vi "Main.vi"() -> ()   [LabVIEW 2012]
uses:
  SprayParams_Array.ctl
  ControlCore_Queue.ctl
  ControlCore_States.ctl
  <vilib>/DAQmx/write.llb/DAQmx Write (Digital Bool 1Line 1Point).vi
  <vilib>/DAQmx/miscellaneous.llb/DAQmx Fill In Error Info.vi
  <userlib>/Utility/ErrorLog_lib.lvlib
panel:
  out "ETF (min)":dbl format="%#.1g"
  out "Progress Bar":dbl(slide) scale=0.0..1.0
  out "String":string
  in  "STOP":bool
  in  "Close":bool
  in  "Open":bool
  in  "Start":bool
  out "Relay Status":bool
  in  "Spray Parameters":T1[](array[typedef])=[{"Cycle#"=20, "Spray Time"=1.25, "Dry Time"=15.0}] caption="Cycle#, Spray Time (s), Dry Time (s)"
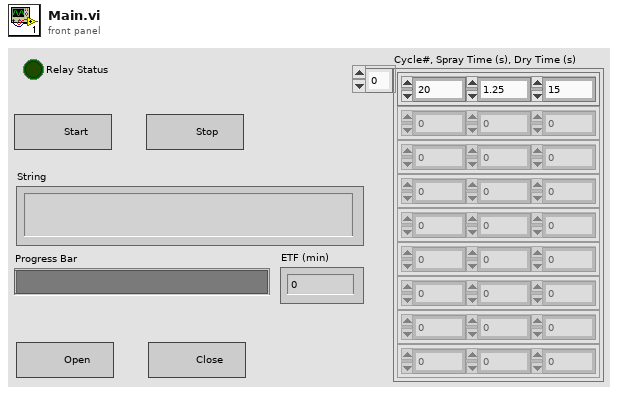
[diagram p1: front panel]
types:
  T1 = typedef "SprayParams_Array.ctl" = cluster{"Cycle#":i32, "Spray Time":dbl, "Dry Time":dbl}
  T2 = typedef "ControlCore_Queue.ctl" = cluster{"State":T3, "Params.":variant}
  T3 = typedef "ControlCore_States.ctl" = enum16{"Initialize", "RunRoutine", "OpenValve", "CloseValve", "_STOP_", "Close", "Quit"}
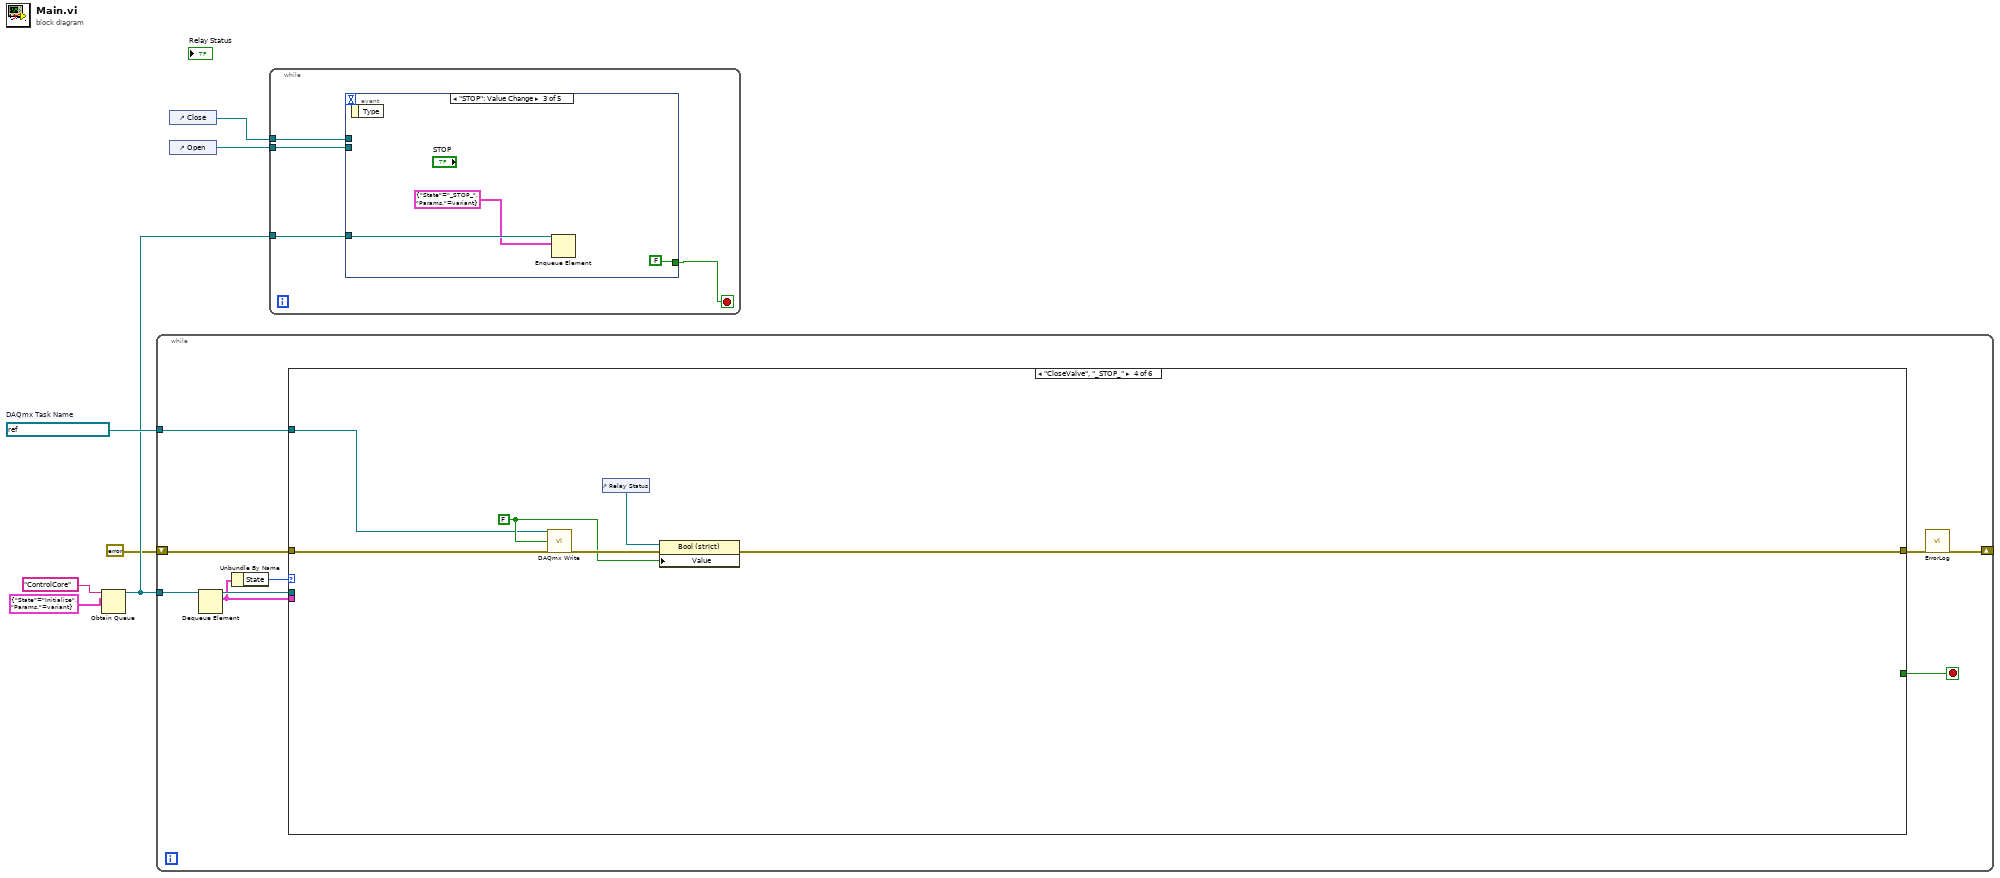
[diagram p0: block diagram]
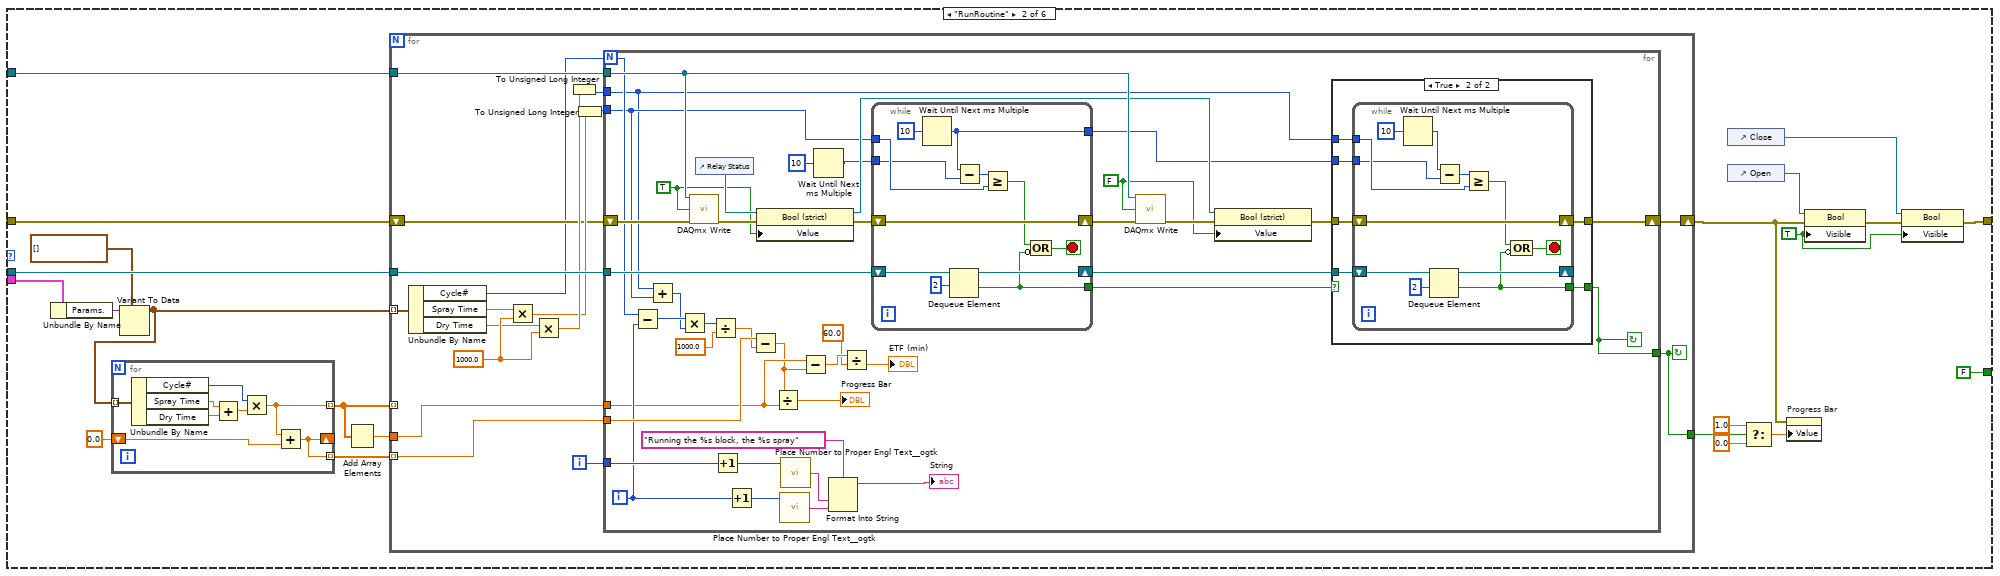
[diagram p3: hidden frame]
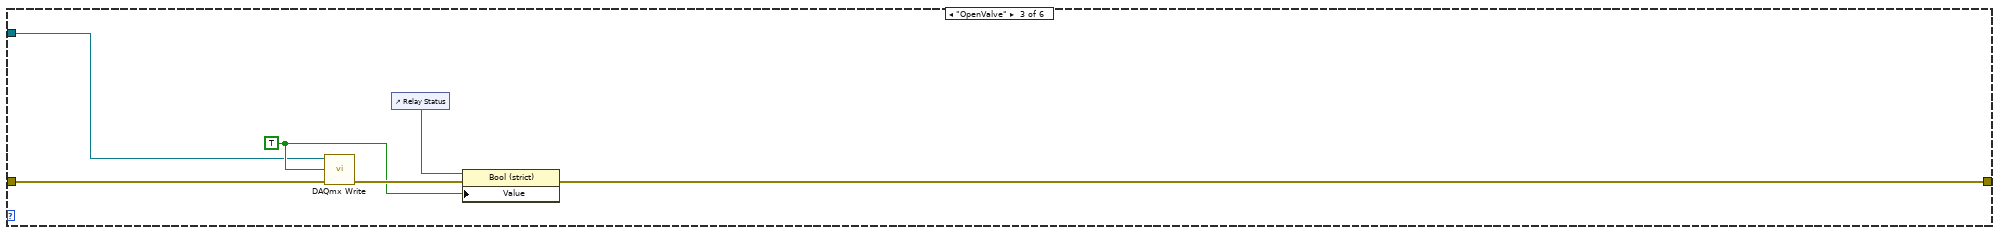
[diagram p5: hidden frame]
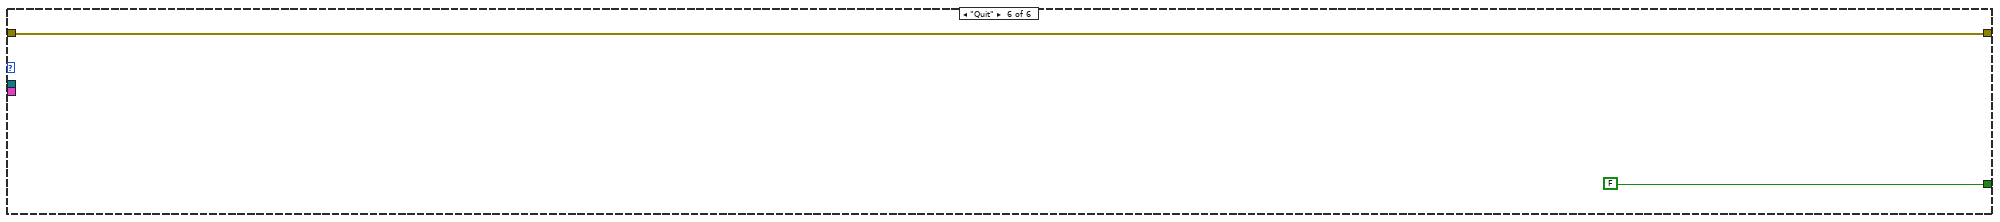
[diagram p7: hidden frame]
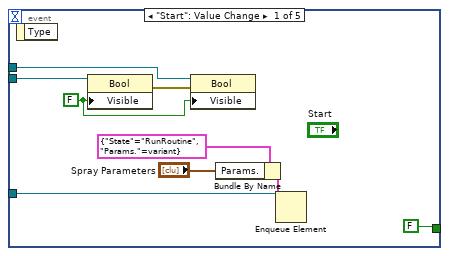
[diagram p8: hidden frame]
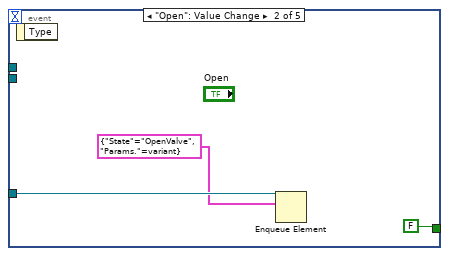
[diagram p9: hidden frame]
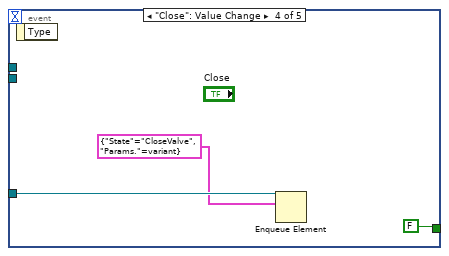
[diagram p10: hidden frame]
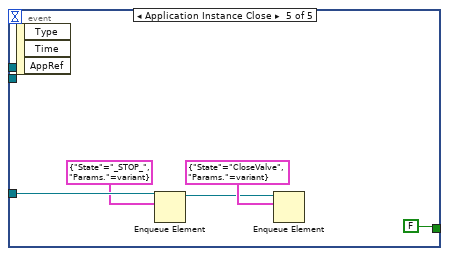
[diagram p11: hidden frame]
diagram:
  w5 = refnum<k21> "RelayOutputControl"  # DAQmx Task Name
  n1 = Obtain Queue(name (unnamed)="ControlCore", element data type=T2 {"State"=enum."Initialize", "Params."=variant}) -> (queue out=w4:refnum<queue>)  [unwired: 3 in, 2 out]
  n2 = while {
    tunnel: w4 -> [w15]
    tunnel: w5 -> [w16]
    shift-right: [w14] -> _
    shift-left: errorcluster {"status"=FALSE, "code"=0, "source"=""} ("error out") -> [w13]
    stop <- w8 stop-if-true
    n3 = Dequeue Element(queue=w15) -> (queue out=w12:refnum<queue>, element=w11:T2)  [unwired: 2 in, 2 out]
    n4 = Unbundle By Name(w11) -> ("State"=w10:T3)
    n5 = case shown="\"CloseValve\", \"_STOP_\"" w10 {
      tunnel: w12 -> [_ w39 _ _ _ _]
      tunnel: w11 -> [_ w38 _ _ _ _]
      tunnel: w16 -> [_ w35 w140 w146 _ _]
      tunnel: w13 -> [w17 w34 w142 w148 w151 w152]
      tunnel: [w17 w19 w139 w145 w151 w152] -> w9
      tunnel: [_ FALSE _ _ _ FALSE] -> w8
      frame "Initialize", Default {
      }
      frame "RunRoutine" {
        w22 = TRUE ("Visible")
        n6 = Unbundle By Name(w38) -> ("Params."=w37:variant)
        n7 = Variant To Data(type=T1[] [], Variant=w37) -> (data=w32:T1[])  [unwired: 1 in, 1 out]
        n8 = for {
          tunnel: w32 -> [w43] mode=indexing
          shift-right: [w41] -> _
          shift-left: 0.0 -> [w42]
          tunnel: [w41] -> w30 mode=indexing
          tunnel: [w40] -> w28 mode=indexing
          n9 = Unbundle By Name(w43) -> ("Cycle#"=w47:i32, "Spray Time"=w45:dbl, "Dry Time"=w44:dbl)
          n10 = Add(x=w45, y=w44) -> (x+y=w46:dbl)
          n11 = Multiply(x=w47, y=w46) -> (x*y=w40:dbl)
          n12 = Add(x=w40, y=w42) -> (x+y=w41:dbl)
        }
        n13 = Add Array Elements(numeric array=w28) -> (sum=w29:dbl)
        n14 = for {
          tunnel: w39 -> [w64]
          tunnel: w32 -> [w63] mode=indexing
          tunnel: w35 -> [w59]
          shift-right: [w57] -> w18
          shift-left: w34 -> [w58]
          tunnel: w30 -> [w50] mode=indexing
          tunnel: w29 -> [w49]
          tunnel: w28 -> [_] mode=indexing
          tunnel: [w48] -> w27
          i -> [w54]
          stop <- w48 continue-if-true
          w60 = 1000.0
          n15 = Unbundle By Name(w63) -> ("Cycle#"=w51:i32, "Spray Time"=w52:dbl, "Dry Time"=w53:dbl)
          n16 = Multiply(x=w52, y=w60) -> (x*y=w61:dbl)
          n17 = Multiply(x=w53, y=w60) -> (x*y=w62:dbl)
          n18 = To Unsigned Long Integer(number=w62) -> (unsigned 32bit integer=w56:u32)
          n19 = To Unsigned Long Integer(number=w61) -> (unsigned 32bit integer=w55:u32)
          n20 = for {
            N: w51 -> [w81]
            shift-right: [w102] -> w57
            shift-left: w58 -> [w104]
            tunnel: w55 -> [w78]
            tunnel: w56 -> [w70]
            tunnel: w64 -> [w103]
            tunnel: w59 -> [w98]
            tunnel: [w88] -> w48
            tunnel: w54 -> [w80]
            tunnel: w49 -> [w68]
            tunnel: w50 -> [w74]
            i -> [w71]
            stop <- w88 continue-if-true
            w92 = FALSE ("data")
            w95 = TRUE ("data")
            n21 = Subtract(x=w81, y=w71) -> (x-y=w79:i32)
            n22 = Add(x=w70, y=w78) -> (x+y=w77:u32)
            n23 = Multiply(x=w79, y=w77) -> (x*y=w76:u32)
            n24 = call-poly <vilib>:"DAQmx Write.vi"("task/channels in"=w98, "data"=w95, "error in"=w104) -> ("error out"=w106:errorcluster)  [unwired: 10 in, 2 out]
            n25 = control-ref of="Relay Status"() -> (w96:refnum<vi>)
            n26 = Divide(x=w76, y=1000.0) -> (x/y=w73:dbl)
            n27 = Increment(x=w80) -> (x+1=w87:i32)
            n28 = Increment(x=w71) -> (x+1=w86:i32)
            n29 = Subtract(x=w74, y=w73) -> (x-y=w67:dbl)
            n30 = property class="Bool (strict)"(reference=w96, error in=w106, "Value"=w95) -> (reference out=w93:refnum<vi>, error out=w97:errorcluster)
            n31 = Divide(x=w67, y=w68) -> (x/y=→"Progress Bar":dbl)
            n32 = call <userlib>:"Place Number to Proper Engl Text__ogtk.vi"("Numeric"=w86) -> ("String"=w85:string)  [unwired: 4 in]
            n33 = call <userlib>:"Place Number to Proper Engl Text__ogtk.vi"("Numeric"=w87) -> ("String"=w84:string)  [unwired: 4 in]
            n34 = Subtract(x=w68, y=w67) -> (x-y=w69:dbl)
            n35 = Wait Until Next ms Multiple(millisecond multiple=u32 10) -> (millisecond timer value=w90:u32)
            n36 = Format Into String(format string="Running the %s block, the %s spray", w84, w85) -> (resulting string=→"String":string)  [unwired: 2 in, 1 out]
            n37 = Divide(x=w69, y=60.0 ("x")) -> (x/y=→"ETF (min)":dbl)
            n38 = while {
              shift-right: [w138] -> w105
              shift-left: w97 -> [w138]
              tunnel: w78 -> [w135]
              shift-right: [w131] -> w101
              shift-left: w103 -> [w132]
              tunnel: [w130] -> w99
              tunnel: w90 -> [w129]
              tunnel: [w128] -> w89
              stop <- w134 stop-if-true
              n39 = Wait Until Next ms Multiple(millisecond multiple=u32 10) -> (millisecond timer value=w128:u32)
              n40 = Dequeue Element(queue=w132, timeout in ms (-1)=2) -> (queue out=w131:refnum<queue>, timed out?=w130:bool)  [unwired: 1 in, 2 out]
              n41 = Subtract(x=w128, y=w129) -> (x-y=w136:u32)
              n42 = Greater Or Equal?(x=w136, y=w135) -> (x >= y?=w133:bool)
              n43 = Compound Arithmetic op=OR(w133, invert w130) -> (w134:bool)
            }
            n44 = call-poly <vilib>:"DAQmx Write.vi"("task/channels in"=w98, "data"=w92, "error in"=w105) -> ("error out"=w100:errorcluster)  [unwired: 10 in, 2 out]
            n45 = property class="Bool (strict)"(reference=w93, error in=w100, "Value"=w92) -> (error out=w94:errorcluster)  [unwired: 1 out]
            n46 = case shown="True" w99 {
              selector: w99 -> [w107 _]
              tunnel: [w108 w114] -> w102
              tunnel: w101 -> [_ w113]
              tunnel: w94 -> [w108 w112]
              tunnel: w89 -> [_ w110]
              tunnel: w70 -> [_ w111]
              tunnel: [w107 w109] -> w88
              frame False {
              }
              frame True {
                n47 = while {
                  shift-right: [w126] -> w114
                  shift-left: w112 -> [w126]
                  tunnel: w111 -> [w122]
                  shift-right: [w118] -> _
                  shift-left: w113 -> [w119]
                  tunnel: [w117] -> w109
                  tunnel: w110 -> [w116]
                  stop <- w121 stop-if-true
                  n48 = Wait Until Next ms Multiple(millisecond multiple=u32 10) -> (millisecond timer value=w124:u32)
                  n49 = Dequeue Element(queue=w119, timeout in ms (-1)=2) -> (queue out=w118:refnum<queue>, timed out?=w117:bool)  [unwired: 1 in, 2 out]
                  n50 = Subtract(x=w124, y=w116) -> (x-y=w123:u32)
                  n51 = Greater Or Equal?(x=w123, y=w122) -> (x >= y?=w120:bool)
                  n52 = Compound Arithmetic op=OR(w120, invert w117) -> (w121:bool)
                }
              }
            }
          }
        }
        n53 = control-ref of="Close"() -> (w20:refnum<vi>)
        n54 = control-ref of="Open"() -> (w21:refnum<vi>)
        n55 = Select(t=1.0, s=w27, f=0.0) -> (s? t:f=w24:dbl)
        n56 = property on="Progress Bar" class="Slide (strict)"(error in=w18, "Value"=w24) -> ()  [unwired: 1 in, 2 out]
        n57 = property class="Bool"(reference=w21, error in=w18, "Visible"=w22) -> (error out=w23:errorcluster)  [unwired: 1 out]
        n58 = property class="Bool"(reference=w20, error in=w23, "Visible"=w22) -> (error out=w19:errorcluster)  [unwired: 1 out]
      }
      frame "OpenValve" {
        w141 = TRUE ("data")
        n59 = call-poly <vilib>:"DAQmx Write.vi"("task/channels in"=w140, "data"=w141, "error in"=w142) -> ("error out"=w144:errorcluster)  [unwired: 10 in, 2 out]
        n60 = control-ref of="Relay Status"() -> (w143:refnum<vi>)
        n61 = property class="Bool (strict)"(reference=w143, error in=w144, "Value"=w141) -> (error out=w139:errorcluster)  [unwired: 1 out]
      }
      frame "CloseValve", "_STOP_" {
        w147 = FALSE ("data")
        n62 = call-poly <vilib>:"DAQmx Write.vi"("task/channels in"=w146, "data"=w147, "error in"=w148) -> ("error out"=w150:errorcluster)  [unwired: 10 in, 2 out]
        n63 = control-ref of="Relay Status"() -> (w149:refnum<vi>)
        n64 = property class="Bool (strict)"(reference=w149, error in=w150, "Value"=w147) -> (error out=w145:errorcluster)  [unwired: 1 out]
      }
      frame "Close" {
      }
      frame "Quit" {
      }
    }
    n65 = call <userlib>:"ErrorLog.vi"("error in (no error)"=w9) -> ("error out"=w14:errorcluster)  [unwired: 10 in]
  }
  n66 = control-ref of="Close"() -> (w1:refnum<vi>)
  n67 = control-ref of="Open"() -> (w2:refnum<vi>)
  n68 = while {
    tunnel: w4 -> [w157]
    tunnel: w2 -> [w155]
    tunnel: w1 -> [w154]
    stop <- w156 stop-if-true
    n69 = event shown="[2] \"STOP\": Value Change" {
      selector: _ -> [_ _ _ _ _]
      dyn-events: _ -> [_ _ _ _ _]
      timeout: _ -> [_ _ _ _ _]
      tunnel: w157 -> [w166 w169 w172 w175 w180]
      tunnel: [FALSE FALSE FALSE FALSE FALSE] -> w156
      tunnel: w155 -> [w161 _ _ _ _]
      tunnel: w154 -> [w160 _ _ _ _]
      event "Start": Value Change {
        w158 = FALSE ("Visible")
        n70 = event-data() -> ()  [unwired: 1 in, 1 out]
        n71 = property class="Bool"(reference=w161, "Visible"=w158) -> (error out=w159:errorcluster)  [unwired: 1 in, 1 out]
        n72 = property class="Bool"(reference=w160, error in=w159, "Visible"=w158) -> ()  [unwired: 2 out]
        n73 = Bundle By Name(cluster=T2 {"State"=enum."RunRoutine", "Params."=variant}, "Params."="Spray Parameters") -> (w165:T2)
        n74 = Enqueue Element(queue=w166, element=w165) -> ()  [unwired: 2 in, 3 out]
      }
      event "Open": Value Change {
        n75 = event-data() -> ()  [unwired: 1 in, 1 out]
        n76 = Enqueue Element(queue=w169, element=T2 {"State"=enum."OpenValve", "Params."=variant}) -> ()  [unwired: 2 in, 3 out]
      }
      event "STOP": Value Change {
        n77 = event-data() -> ()  [unwired: 1 in, 1 out]
        n78 = Enqueue Element(queue=w172, element=T2 {"State"=enum."_STOP_", "Params."=variant}) -> ()  [unwired: 2 in, 3 out]
      }
      event "Close": Value Change {
        n79 = event-data() -> ()  [unwired: 1 in, 1 out]
        n80 = Enqueue Element(queue=w175, element=T2 {"State"=enum."CloseValve", "Params."=variant}) -> ()  [unwired: 2 in, 3 out]
      }
      event Application Instance Close {
        n81 = event-data() -> ()  [unwired: 1 in, 3 out]
        n82 = Enqueue Element(queue=w180, element=T2 {"State"=enum."_STOP_", "Params."=variant}) -> (queue out=w176:refnum<queue>)  [unwired: 2 in, 2 out]
        n83 = Enqueue Element(queue=w176, element=T2 {"State"=enum."CloseValve", "Params."=variant}) -> ()  [unwired: 2 in, 3 out]
      }
    }
  }
